vi "Write.vi"(8 "error in (no error)":errorcluster, 9 "timeout ms (25000)":i32, 10 "data in":string, 11 "connection ID":refnum<k5>) -> (0 "error out":errorcluster, 3 "connection ID out":refnum<k5>)   [LabVIEW 2020]
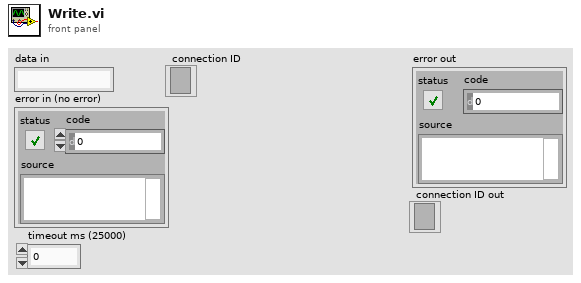
[diagram p1: front panel]
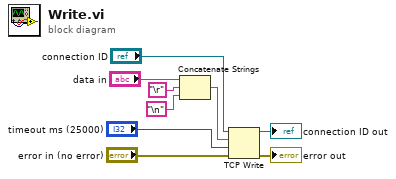
[diagram p0: block diagram]
diagram:
  n1 = Concatenate Strings("data in", "\r", "\n") -> (w5:string)
  n2 = TCP Write(connection ID="connection ID", data in=w5, error in (no error)="error in (no error)", 9:"timeout ms (25000)") -> (connection ID out=→"connection ID out":refnum<k5>, error out=→"error out":errorcluster)  [unwired: 1 out]
